vi "AlliGator Load Dataset or Series.vi"(4 "Save Phasor Plot with Overlay":bool, 6 "Save Image with Overlay":bool, 7 "VI in":refnum<vi>, 8 "error in (no error)":errorcluster, 9 "Type of Displayed Image":T1 caption="Displayed Image", 10 "File/Folder Path":path, 11 "AlliGator Ctrl Refnums":T2) -> (0 "error out":errorcluster, 1 "Message":string, 3 "AlliGator Q Elements out":T10[](array[typedef]))   [LabVIEW 2021, in "AlliGator Files.lvlib"]
doc: "Detects type of file loaded and generates the series of actions needed to load it."
uses:
  AlliGator Files.lvlib
  AlliGator Q Element.ctl
  AlliGator Q Event.ctl
  AlliGator Ctrl Refnums.ctl
  AlliGator Other Ctrl Refnums.ctl
  AlliGator State Indicator.ctl
  AlliGator Phasor Plot Ctrl Refnums.ctl
  AlliGator Phasor Graph Ctrl Refnums.ctl
  Phasor/Phasor Calibration Type.ctl
  AlliGator Dataset Ctrl Refnums.ctl
  AlliGator Displayed Image.ctl
  AlliGator Registered Events Ctrl Refnums.ctl
  AlliGator Image Histogram Control Refnums.ctl
  Histograms/Linear Histogram Options.ctl
  Histograms/Histogram Bin Option.ctl
  Histograms/Histogram Bin Position.ctl
  AlliGator Decay Fit Map Control Refnums.ctl
  Fits/IRF(X)PSED/Decay Fit Parameters & Derived Quantities List.ctl
  AlliGator FLI Dataset Type.ctl
  Files/Load-Save File Info.ctl
  AlliGator ROI Manager Actions.ctl
  AlliGator Select Folder Mode.ctl
  AlliGator Folder Selection.ctl
  <vilib>/Utility/error.llb/Error Cluster From Error Code.vi
  AlliGator Source Image ROI Storage [SGL] v3.vi
  <userlib>/_OpenG.lib/array/array.llb/Filter 1D Array with Scalar (String)__ogtk.vi
  <vilib>/ErrorRing/Error Ring.xnode
  AlliGator HDF5.lvlib
  <userlib>/_OpenG.lib/file/file.llb/openg_file.lvlib
  Files/Files.lvlib
  Image/Image.lvlib
  AlliGator Action Engine.lvlib
  <userlib>/_OpenG.lib/array/array.llb/openg_array.lvlib
  AlliGator ROIs.lvlib
  Graphs/XY Graph/XY Graph Add-Ons.lvlib
  AlliGator Globals, Variables & Constants.lvlib
  AlliGator Scripts.lvlib
  AlliGator Decay Fit Parameter Map.lvlib
  GUI/GUI.lvlib
  AlliGator Settings.lvlib
  Sound/Sound.lvlib
  AlliGator Source Image.lvlib
  AlliGator GUI.lvlib
  Phasor/Phasor.lvlib
  Histograms/Histogram Window.lvlib
  Fits/Fits.lvlib
panel:
  out "Script out":bool
  in  "Script in":bool
  # "see the AlliGator License on the block diagram (Ctrl+E or Window:Show Block Diagram)"
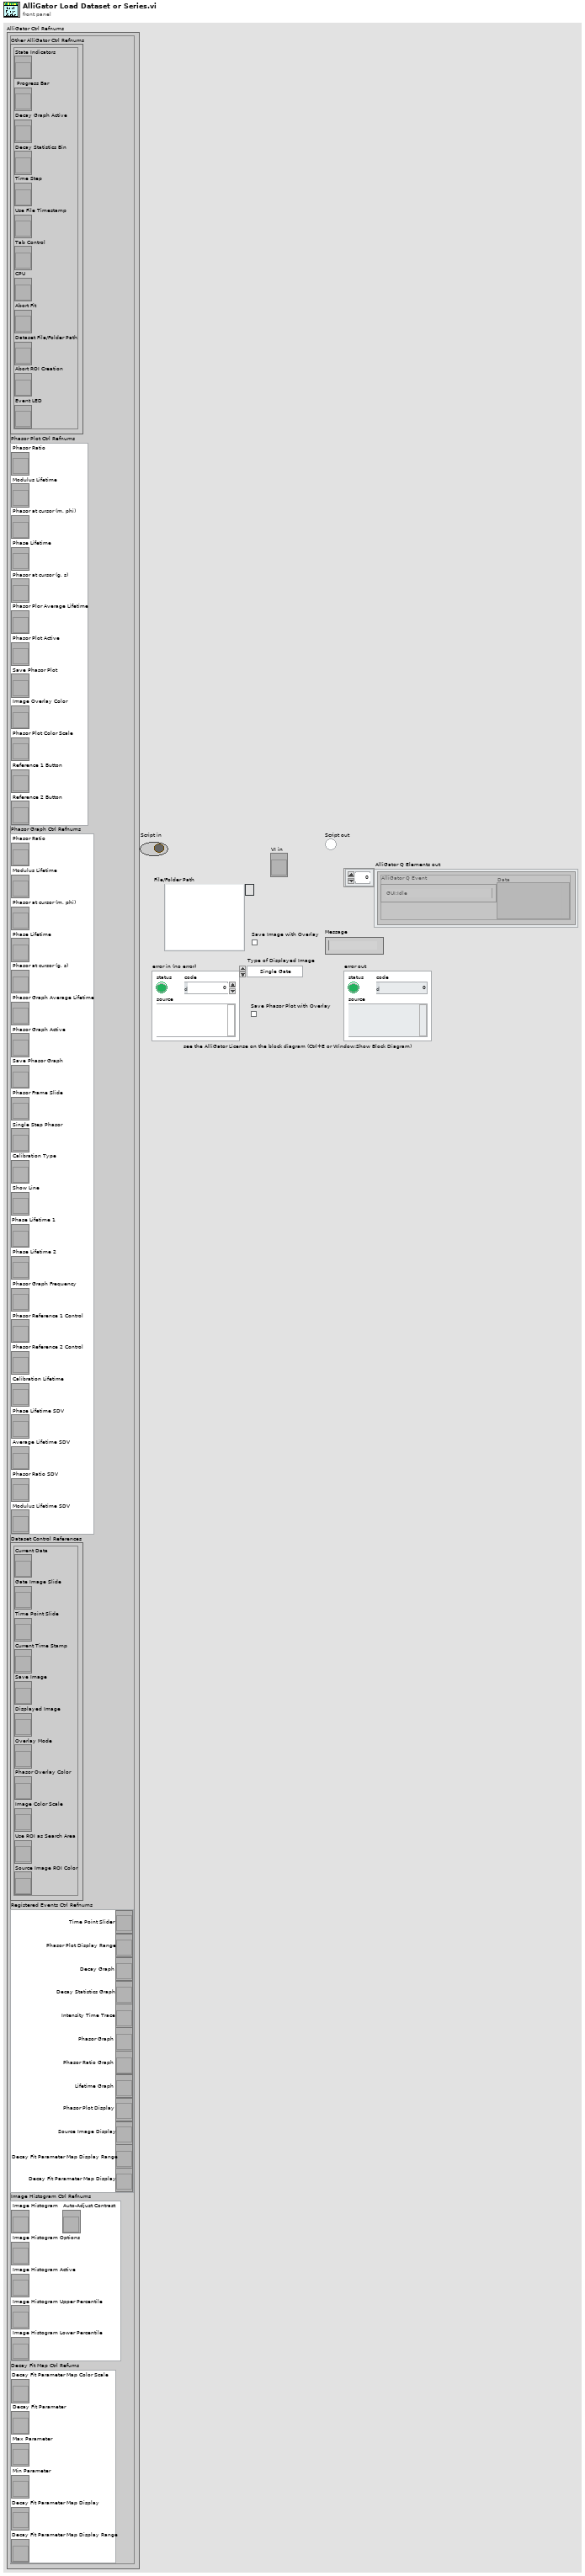
[diagram p1: front panel]
types:
  T1 = typedef "AlliGator Source Image.lvlib/AlliGator Displayed Image.ctl" = enum16{"Single Gate", "Sum of All Gates", "Max of All Gates", "Min of All Gates", "-", "White Ligth Image", "Mask Image"}
  T2 = typedef "AlliGator GUI.lvlib/AlliGator Ctrl Refnums.ctl" = cluster{"Other AlliGator Ctrl Refnums":T3, "Phasor Plot Ctrl Refnums":T4, "Phasor Graph Ctrl Refnums":T5, "Dataset Control References":T6, "Registered Events Ctrl Refnums":T7, "Image Histogram Ctrl Refnums":T8, "Decay Fit Map Ctrl Refums":T9}
  T3 = typedef "AlliGator GUI.lvlib/AlliGator Other Ctrl Refnums.ctl" = cluster{"State Indicators":refnum<vi>, " Progress Bar":refnum<vi>, "Decay Graph Active":refnum<vi>, "Decay Statistics Bin":refnum<vi>, "Time Step":refnum<vi>, "Use File Timestamp":refnum<vi>, "Tab Control":refnum<vi>, "CPU":refnum<vi>, "Abort Fit":refnum<vi>, "Dataset File/Folder Path":refnum<vi>, "Abort ROI Creation":refnum<vi>, "Event LED":refnum<vi>}
  T4 = typedef "AlliGator GUI.lvlib/AlliGator Phasor Plot Ctrl Refnums.ctl" = cluster{"Phasor Ratio":refnum<vi>, "Modulus Lifetime":refnum<vi>, "Phasor at cursor (m, phi)":refnum<vi>, "Phase Lifetime":refnum<vi>, "Phasor at cursor (g, s)":refnum<vi>, "Phasor Plor Average Lifetime":refnum<vi>, "Phasor Plot Active":refnum<vi>, "Save Phasor Plot":refnum<vi>, "Image Overlay Color":refnum<vi>, "Phasor Plot Color Scale":refnum<vi>, "Reference 1 Button":refnum<vi>, "Reference 2 Button":refnum<vi>}
  T5 = typedef "AlliGator GUI.lvlib/AlliGator Phasor Graph Ctrl Refnums.ctl" = cluster{"Phasor Ratio":refnum<vi>, "Modulus Lifetime":refnum<vi>, "Phasor at cursor (m, phi)":refnum<vi>, "Phase Lifetime":refnum<vi>, "Phasor at cursor (g, s)":refnum<vi>, "Phasor Graph Average Lifetime":refnum<vi>, "Phasor Graph Active":refnum<vi>, "Save Phasor Graph":refnum<vi>, "Phasor Frame Slide":refnum<vi>, "Single Step Phasor":refnum<vi>, "Calibration Type":refnum<vi>, "Show Line":refnum<vi>, "Phase Lifetime 1":refnum<vi>, "Phase Lifetime 2":refnum<vi>, "Phasor Graph Frequency":refnum<vi>, "Phasor Reference 1 Control":refnum<vi>, "Phasor Reference 2 Control":refnum<vi>, "Calibration Lifetime":refnum<vi>, "Phase Lifetime SDV":refnum<vi>, "Average Lifetime SDV":refnum<vi>, "Phasor Ratio SDV":refnum<vi>, "Modulus Lifetime SDV":refnum<vi>}
  T6 = typedef "AlliGator GUI.lvlib/AlliGator Dataset Ctrl Refnums.ctl" = cluster{"Current Data":refnum<vi>, "Gate Image Slide":refnum<vi>, "Time Point Slide":refnum<vi>, "Current Time Stamp":refnum<vi>, "Save Image":refnum<vi>, "Displayed Image":refnum<vi>, "Overlay Mode":refnum<vi>, "Phasor Overlay Color":refnum<vi>, "Image Color Scale":refnum<vi>, "Use ROI as Search Area":refnum<vi>, "Source Image ROI Color":refnum<vi>}
  T7 = typedef "AlliGator GUI.lvlib/AlliGator Registered Events Ctrl Refnums.ctl" = cluster{"Time Point Slider":refnum<vi>, "Phasor Plot Display Range":refnum<vi>, "Decay Graph":refnum<vi>, "Decay Statistics Graph":refnum<vi>, "Intensity Time Trace":refnum<vi>, "Phasor Graph":refnum<vi>, "Phasor Ratio Graph":refnum<vi>, "Lifetime Graph":refnum<vi>, "Phasor Plot Display":refnum<vi>, "Source Image Display":refnum<vi>, "Decay Fit Parameter Map Display Range":refnum<vi>, "Decay Fit Parameter Map Display":refnum<vi>}
  T8 = typedef "AlliGator GUI.lvlib/AlliGator Image Histogram Control Refnums.ctl" = cluster{"Image Histogram":refnum<vi>, "Image Histogram Options":refnum<vi>, "Image Histogram Active":refnum<vi>, "Image Histogram Upper Percentile":refnum<vi>, "Image Histogram Lower Percentile":refnum<vi>, "Auto-Adjust Contrast":refnum<vi>}
  T9 = typedef "AlliGator Decay Fit Parameter Map.lvlib/AlliGator Decay Fit Map Control Refnums.ctl" = cluster{"Decay Fit Parameter Map Color Scale":refnum<vi>, "Decay Fit Parameter":refnum<vi>, "Max Parameter":refnum<vi>, "Min Parameter":refnum<vi>, "Decay Fit Parameter Map Display":refnum<vi>, "Decay Fit Parameter Map Display Range":refnum<vi>}
  T10 = typedef "AlliGator Action Engine.lvlib/AlliGator Q Element.ctl" = cluster{"AlliGator Q Event":T11, "Data":variant}
  T11 = typedef "AlliGator Action Engine.lvlib/AlliGator Q Event.ctl" = enum16{"---- Files ----", "Files:Set Batch Export Files To Save", "Files:Set Dataset Loading & Pre-processing Options", "Files:Check #Frames in Dataset", "Files:Increment Frame Index", "Files:Open Mask Image", "Files:Open White Light Image", "Files:Open Single Dataset", "Files:New Folder of Folders Selected", "Files:Load File (all Types)_Scriptable", "Files:Move Flattened Series to Folders Series", "Files:Select Folder", "Files:Load FLI Dataset", "Files:Load Swiss SPAD 1 Dataset", "Files:Load Swiss SPAD 2 Dataset", "Files:Load .sdt FLI Dataset", "Files:Load .ptu FLI Dataset", "Files:Load .bin FLI Dataset", "Files:Load Single Gate Image Folder", "Files:Load I/m/phi Dataset (deprecated)", "Files:Load Single Image", "Files:Subtract Background File", "Files:Export FLI Dataset", "Files:Load HDF5 FLI Dataset", "Files:Set Destination File Path", "Files:Save Mask Image", "Files:Batch Conversion", "Files:New Folder Selected", "Files:Close FLI Dataset", "Files:Close FLI Dataset Series", "Files:Close White Light Image", "Files:Close Mask Image", "---- FLI Dataset ----", "FLI Dataset:Channel Arithmetic", "FLI Dataset:Export Average Lifetime Map as ASCII", "FLI Dataset:Export User-Defined Quantity Map as ASCII", "FLI Dataset:Python Function FLI Dataset Event", "FLI Dataset:ROI Analysis", "FLI Dataset:Tilted Logistic Square Gated IRF Characteristics Map", "FLI Dataset:Logistic Square Gated IRF Characteristics Map", "FLI Dataset:Square Gated IRF Characteristics Map", "FLI Dataset:Multi-ROI Single-Pixel Phasor Analysis", "FLI Dataset:Multi-ROI Single-Pixel NLSF Analysis", "FLI Dataset:All ROIs IRF Extraction", "FLI Dataset:All ROIs Decay Fit Non-Interactive (Fast + Individual IRF)", "FLI Dataset:All ROIs Phasor Analysis", "FLI Dataset:All ROIs Decay Fit", "FLI Dataset:Fluorescence Decay Statistics", "FLI Dataset:Update Decay Statistics Graph", "FLI Dataset:Get Decay from ROI", "FLI Dataset:All ROIs Average Lifetimes", "---- FLI Dataset Series ----", "FLI Dataset Series:Sum All Datasets in Series", "FLI Dataset Series:Add Dataset to Accumulated Dataset", "FLI Dataset Series:Display Accumulated Dataset", "FLI Dataset Series:Clear Dataset Series Sum", "FLI Dataset Series:Time-Series Analysis (NLSF)", "FLI Dataset Series:Time-Series Analysis (Phasor)", "---- Image ----", "Image:Update Image Profile Plots", "Image:Image Histogram Cursor Move", "Image:Image Histogram", "Image:Image Contrast", "Image:Set Image Histogram Cursor Move Flag", "Image:Clear Image Overlay", "Image:Use ROI as Search Area", "Image:Set ROI Diameter", "Image:Save Image Data as TIFF", "Image:Save Displayed Image with Overlay", "Image:Save Image Overlay Only", "Image:Save Image as Hot Pixel Mask", "Image:Change Source Image Color Palette", "Image:Copy Image to Clipboard", "Image:Source Image ROI Selection", "Image:Delete All ROIs", "Image:Delete All Unselected ROIs", "Image:Delete ROI", "Image:Merge All ROIs", "Image:Store ROI", "Image:Source Image ROI Storage", "Image:Export ROI Description to Notebook", "Image:Save ROI", "Image:Load ROI", "Image:Paste ROI Definition", "Image:Clear ROI", "Image:Identify ROIs in Mask Image", "Image:Create Complementary ROI", "Image:Create Contour ROI", "Image:Create ROI(s) from Pixels with Peak above Min_Scriptable", "Image:Create ROI(s) from Pixels with Intensity above Min_Scriptable", "Image:Compute ROI Statistics", "Image:Delete ROI(s) based on ROI Characteristics", "Image:Create ROI Grid", "Image:ROI to Individual Pixel ROIs", "Image:Python Function Source Image Event", "Image:Show Phasor Calibration Map ROI Centers", "Image:Convert ROI to Mask Image", "Image:Mouse Move", "Image:Mouse Up", "Image:Set Source Image Mouse Move Flag", "Image:Add Scale Bar Overlay", "Image:Delete Existing ROIs Option", "---- Decay ----", "Decay:Clear IRF/Reference Plot", "Decay:Clear Local IRFs", "Decay:Add Decay to Graph", "Decay:Smoothen Plot", "Decay:Smoothen Plot Tail", "Decay:Average Selected Plots", "Decay:Extract IRF", "Decay:Optimal IRF Extraction", "Decay:Threshold IRF", "Decay:Fit to Model IRF", "Decay:Fit IRF to Square Gate", "Decay:Fit IRF to Logistic Square Gate", "Decay:Fit IRF to Tilted Logistic Square Gate", "Decay:Create Bounding Cursors Set", "Decay:Export Bounding Cursors Definition to Notebook", "Decay:Denoise Plot", "Decay:Compute Cumulative Function", "Decay:Use as Reference Decay", "Decay:Show Reference Decay/IRF", "Decay:Extrapolate Decay", "Decay:Create Head & Tail Bounding Cursors", "Decay:Store Cursor-defined Head & Tail Fractions", "Decay:Rebin Plot", "Decay:1-Normalize Decay", "Decay:[0-1]-Normalize Plot", "Decay:Straighten Decay", "Decay:Shift Decay", "Decay:Fold Decay", "Decay:Fit Decay", "Decay:Global Fit of Selected Decays", "Decay:Post Global Fit Script", "Decay:Add Global Fit Parameters to Graph", "Decay:Add Decay Parameter(s) to Plot (Graph)", "Decay:Export Decay to Phasor Graph", "Decay:Plot Decay Shifts", "Decay:Compute Average Lifetime", "Decay:Plot Convolution", "Decay:Graph Tip Strip Update", "---- Decay Statistics ----", "Decay Statistics:Tip Strip Update", "---- Intensity Time Trace ----", "Intensity Time Trace:Use File Timestamp", "Intensity Time Trace:Load Intensity Corrections File", "Intensity Time Trace:Clear Intensity Corrections File", "Intensity Time Trace:Tip Strip Update", "---- Phasor Plot ----", "Phasor Plot:Build Phasor Plot", "Phasor Plot:Change Phasor Plot Color Palette", "Phasor Plot:Adjust Phasor Plot Display Range", "Phasor Plot:Highlight Image ROI in Phasor Plot", "Phasor Plot:Save Phasor Plot Image with Overlay", "Phasor Plot:Export Complex Phasor Map", "Phasor Plot:Export Phasor Ratio Map", "Phasor Plot:Export Average Lifetime Map", "Phasor Plot:Compute Phase Lifetime Histogram", "Phasor Plot:Compute Phasor Ratio Histogram", "Phasor Plot:Compute Phase Lifetime vs Intensity Scatter Plot", "Phasor Plot:Weber 2-Component Decomposition", "Phasor Plot:Update Phasor Color Map Vertices", "Phasor Plot:Clear Phasor Overlay", "Phasor Plot:Use Segment Extremities as References", "Phasor Plot:Use UC/Segment Intersections as References", "Phasor Plot:Use UC/Principal Axis Intersections as References", "Phasor Plot:Use UC/Linear Fit Intersections as References", "Phasor Plot:Update Phasor Plot Reference", "Phasor Plot:Show Local Phasor Info in Phasor Plot", "Phasor Plot:Update Phasor Plot State", "Phasor Plot:Phasor Plot ROI Storage", "Phasor Plot:Phasor Plot ROI Selection", "Phasor Plot:Python Function Phasor Plot Event", "Phasor Plot:Overlay Phasor ROI, Ratio or Map in Source Image", "Phasor Plot:Compute Decay of Selected Phasors", "Phasor Plot:Phasor at Image Pixel", "Phasor Plot:Mouse Move", "Phasor Plot:Mouse Up", "Phasor Plot:Display Range Mouse Move", "Phasor Plot:Set Mouse Move Flag", "---- Phasor Graph ----", "Phasor Graph:Calibrated Phasor Map Series", "Phasor Graph:Whole Image Phasor Scatter Plot (Todo)", "Phasor Graph:Get Phasor Value", "Phasor Graph:Create New Phasor Plot Dialog", "Phasor Graph:Update Last Phasor Value", "Phasor Graph:Update Phasor (m, phi)", "Phasor Graph:Remove Single Phasor from Plot", "Phasor Graph:Add Single Phasor to Plot", "Phasor Graph:Remove Phasor Plot", "Phasor Graph:Remove Selected Phasor Plots", "Phasor Graph:Clear Phasor Data", "Phasor Graph:Clear Phasor Graph", "Phasor Graph:Cursor Move", "Phasor Graph:Draw Cursor Connecting Line", "Phasor Graph:Clear Cursor Connecting Line", "Phasor Graph:Find UC Intersection", "Phasor Graph:Use UC/Cursor-Defined Line Intersections", "Phasor Graph:Use Selected Plots Fitted Line/UC Intersections", "Phasor Graph:Use Selected Plots Principal Axis/UC Intersections", "Phasor Graph:Show Single Phasor", "Phasor Graph:Save Single Phasor Plot", "Phasor Graph:Save All Phasor Plots", "Phasor Graph:Load Phasor Plot(s)", "Phasor Graph:Phasor Multiplication", "Phasor Graph:Compute Average Phasor", "Phasor Graph:Compute Multiple Average Phasors (Selected Plots)", "Phasor Graph:Export Single Phasor Plot Phase Lifetimes", "Phasor Graph:Phase Lifetime Trajectory", "Phasor Graph:Phase Lifetime vs Intensity Scatter Plot (deprecated)", "Phasor Graph:Parameter 2 vs Parameter 1 Scatter Plot", "Phasor Graph:Use Cursor n Location", "Phasor Graph:Set Reference n to Current Phase Lifetime Value", "Phasor Graph:Set Reference n to Lifetime Value", "Phasor Graph:Set Cursor n Location", "Phasor Graph:Save Phasor Graph Image", "Phasor Graph:Update SEPL Plot", "Phasor Graph:Export Single Phasor Plot Data", "Phasor Graph:Export Selected Phasor Plots Data", "Phasor Graph:Python Function Phasor Graph Event", "Phasor Graph:Tip Strip Update", "---- Calibration ----", "Calibration:Set Calibration Type", "Calibration:Load/Save Phasor Calibration", "Calibration:Load/Save Phasor Calibration Series", "Calibration:Load/Save Phasor Calibration Map", "Calibration:Use as Calibration", "Calibration:Compute Optimal Calibration from Phasor References", "Calibration:Clear Phasor Calibration", "Calibration:Use as Calibration Series", "Calibration:Use as Calibration Map", "Calibration:Clear Calibration Series", "Calibration:Clear Calibration Map", "Calibration:Apply Phasor Calibration", "Calibration:Update Single Plot Calibration", "Calibration:Update Multiple Plots Calibration", "Calibration:Clear Single Plot Calibration", "Calibration:Clear All Plots Calibrations", "Calibration:Clear Plot(s) Calibration(s)?", "Calibration:Phasor Calibration Maps (# Gates Series)", "---- Phasor Ratio ----", "Phasor Ratio:Clear Reference n", "Phasor Ratio:Toggle Selected Plot(s)  Lock to Reference 1", "Phasor Ratio:Use as Reference n", "Phasor Ratio:Send Reference n to Notebook", "Phasor Ratio:Toggle Selected Plot(s)  Lock to Reference 2", "Phasor Ratio:Compute Phasor Ratio at Mouse Location", "Phasor Ratio:Compute Phasor Plot's Average Phasor Ratio", "Phasor Ratio:Compute Time-Series Phasor Ratios", "Phasor Ratio:Fit Line to Phasor Ratio Plot", "Phasor Ratio:Save References", "Phasor Ratio:Load References", "Phasor Ratio:Update Phasor Reference 1", "Phasor Ratio:Update Phasor Reference 2", "Phasor Ratio:Move Cursor n to Reference n", "Phasor Ratio:Use as Phasor Reference 1 Lifetime", "Phasor Ratio:Use as Phasor Reference 2 Lifetime", "Phasor Ratio:Export Phasor Ratio Map as ASCII", "Phasor Ratio:Tip Strip Update", "---- Lifetime & Other Parameters Graph ----", "Lifetime:Tip Strip Update", "---- Decay Fit Parameter Map ----", "Decay Fit Parameter Map:Export ROI NLSF Data as ASCII", "Decay Fit Parameter Map:Set Decay Fit  Parameter Map Selection", "Decay Fit Parameter Map:Build Decay Fit Parameter Map", "Decay Fit Parameter Map:Change Decay Fit Parameter Map Color Palette", "Decay Fit Parameter Map:Export Decay Fit Parameter Map Data as ASCII", "Decay Fit Parameter Map:Export All Decay Fit Parameter Maps Data as ASCII", "Decay Fit Parameter Map:Send Map Data to Lifetime Graph", "Decay Fit Parameter Map:Save Decay Fit Parameter Map Image", "Decay Fit Parameter Map:Save-Load IRFs & Fit Data", "Decay Fit Parameter Map:Update Local Decay Plots", "Decay Fit Parameter Map:Python Function Decay Fit Parameters Map Event", "Decay Fit Parameter Map:Overlay Decay Fit Parameter Map in Source Image", "Decay Fit Parameter Map:Plot Map Data vs Intensity", "Decay Fit Parameter Map:Mouse Up", "Decay Fit Parameter Map:Display Range Mouse Move", "---- Generic Graph ----", "Generic Graph:Generic XY Graph Event", "Generic Graph:Python Function XY Graph Event", "Generic Graph:New Plot", "Generic Graph:Save Plot", "Generic Graph:XY Plot Histogram", "Generic Graph:Set XY Graph Plot Name", "Generic Graph:Set Last Cursor Style", "Generic Graph:Tip Strip Update", "---- GUI ----", "GUI:Start Script", "GUI:Type of Displayed Image Changed", "GUI:Gate Image Slide Changed", "GUI:Show Busy Icon", "GUI:Show Busy Icon & Abort Button", "GUI:Hide Busy Icon", "GUI:Hide Busy Icon & Abort Button", "GUI:Abort", "GUI:End Script", "GUI:Start Timing", "GUI:End Timing", "GUI:Set State Indicator", "GUI:Send Parameters JSON Strings to Clipboard", "GUI:Set Gate Step", "GUI:Idle", "GUI:Initialization", "GUI:Quit", "GUI:Increment Dataset Index", "GUI:Set Dataset Index to -1", "GUI:Time Series Slider Moved", "GUI:Time Series Slider Changed", "GUI:Toggle Playback or Loop", "GUI:Playback Script", "GUI:Set Phasor Frequency", "GUI:Open Window", "DEBUG"}
  T12 = typedef "AlliGator Files.lvlib/AlliGator FLI Dataset Type.ctl" = enum16{"HDF5 FLI Dataset", "Gate Image Folder", ".sdt FLI Dataset (Becker & Hickl)", ".ptu FLI Dataset (PicoQuant)", "SS1 FLI Dataset", "SS2 FLI Dataset", "I/m/phi Dataset", ".bin FLI Dataset (PicoQuant Binned)", ".bin FLI Dataset (Piccolo Binned)"}
  T13 = typedef "Files.lvlib/Load-Save File Info.ctl" = cluster{"Load/Save":bool, "File Path":path}
  T14 = typedef "ROI Descriptor" = cluster{"Global Rectangle":i32[], "Contours":cluster{"ID":enum32{"External", "Internal"}, "Type":u32, "Coordinates":i32[]}[]}
  T15 = typedef "AlliGator ROIs.lvlib/AlliGator ROI Manager Actions.ctl" = enum16{"Undefined", "Delete Current ROI", "Delete All Unselected ROIs", "Delete Multiple ROIs", "Delete All ROIs", "Swap ROIs", "Insert ROI", "Update Current ROI Descriptor", "Rename Current ROI", "Store New ROI", "Store Multiple ROIs", "Select Next ROI", "Select Previous ROI", "Find Selected ROI", "Show All ROIs", "Update ROI Manager Window", "Merge All ROIs", "Unmerge ROI", "Set Selected ROI by ID"}
  T16 = typedef "AlliGator Files.lvlib/AlliGator Folder Selection.ctl" = cluster{"Folder Selection Mode":T17, "Folder Path":path}
  T17 = typedef "AlliGator Files.lvlib/AlliGator Select Folder Mode.ctl" = enum16{"Select Gate Folder", "Select Folder of Gate Folders", "Select Folder of SwissSPAD 2 Datasets", "Select Folder of .sdt FLI Datasets (Becker & Hickl)", "Select Folder of .ptu FLI Datasets (PicoQuant)", "Select Folder of .bin FLI Datasets (PicoQuant Binned)", "Select Folder of .bin FLI Datasets (Piccolo Binned)", "Select Folder of HDF5 FLI Datasets"}
  T18 = typedef "Image Type" = u32
  T19 = typedef "Fits.lvlib/3-Button Dialog Output.ctl" = enum16{"Window Close", "Button 1", "Button 2", "Button 3"}
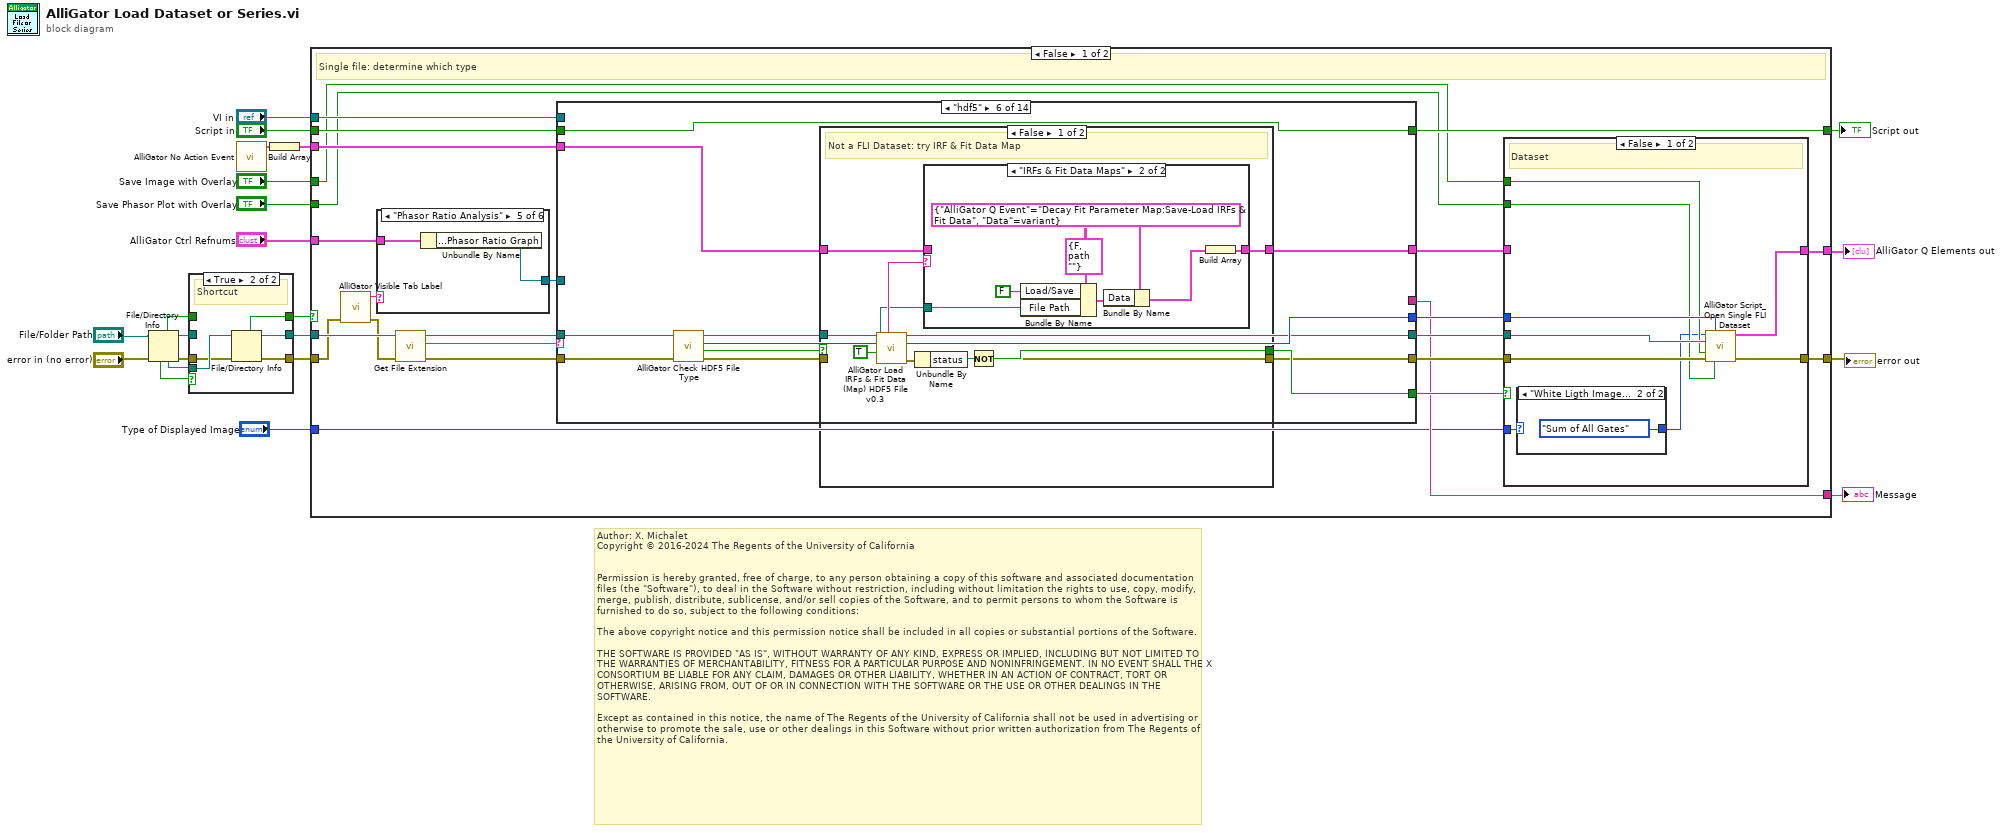
[diagram p0: block diagram]
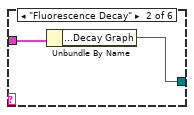
[diagram p3: hidden frame]
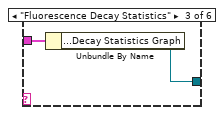
[diagram p4: hidden frame]
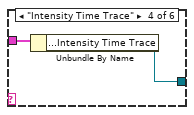
[diagram p5: hidden frame]
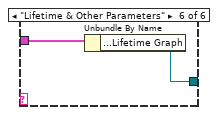
[diagram p6: hidden frame]
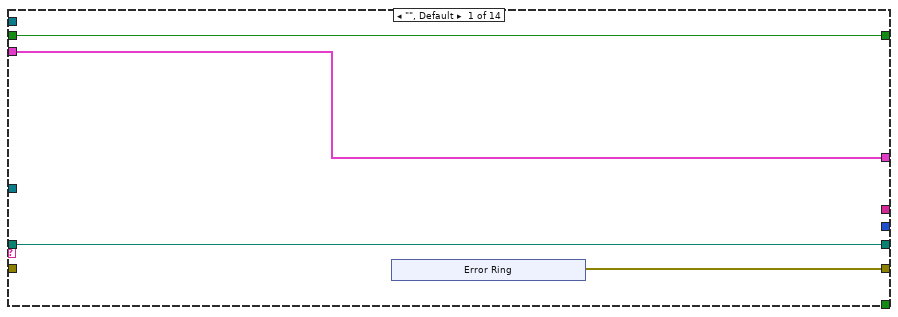
[diagram p9: hidden frame]
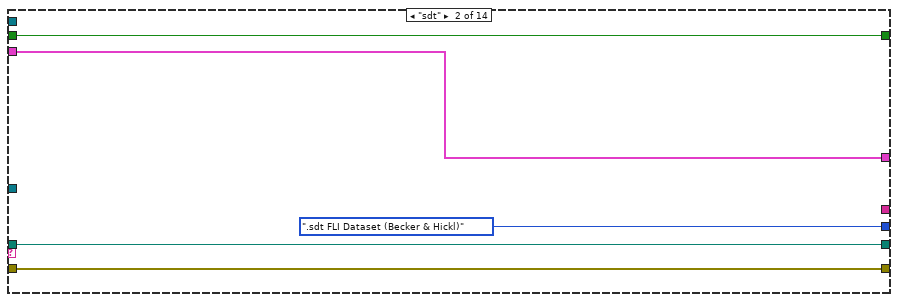
[diagram p10: hidden frame]
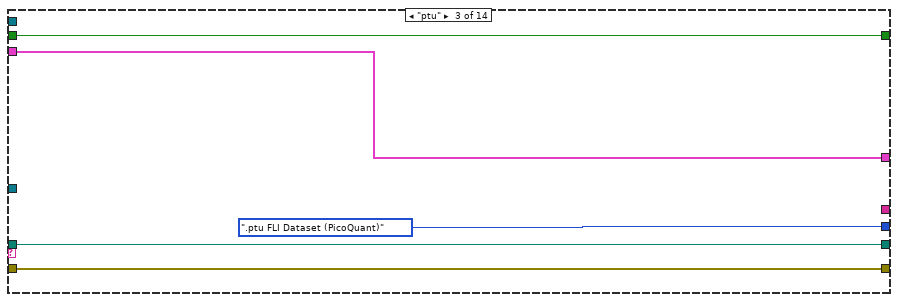
[diagram p11: hidden frame]
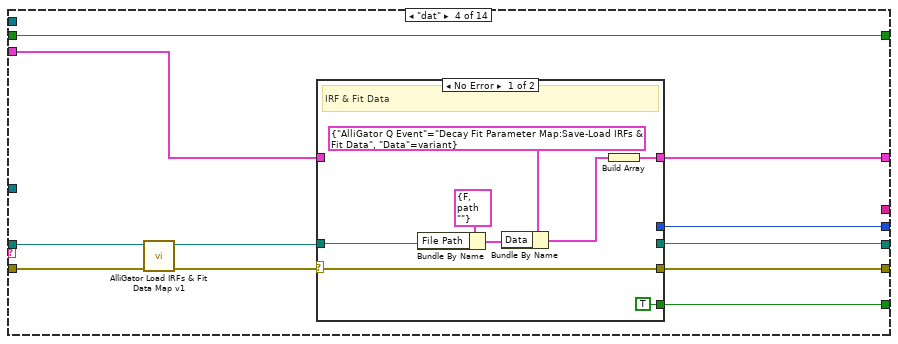
[diagram p12: hidden frame]
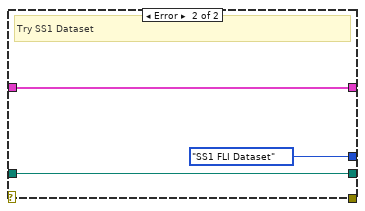
[diagram p13: hidden frame]
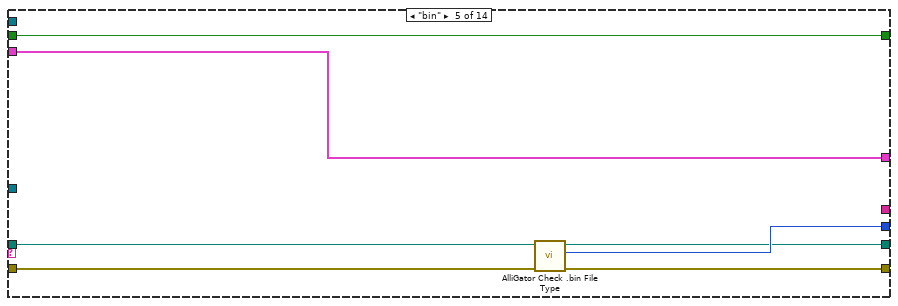
[diagram p14: hidden frame]
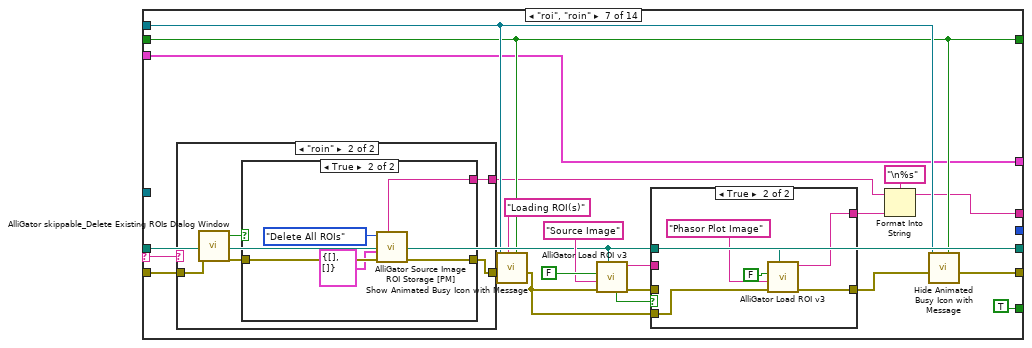
[diagram p17: hidden frame]
diagram:
  # "Author: X. Michalet\nCopyright © 2016-2024 The Regents of the University of California\n \n\nPermission is hereby granted, free of charge, to any person obtaining a copy of this software and associated documentation files (the \"Software\"), to deal in the Software without restriction, including without limitation the rights to use, copy, modify, merge, publish, distribute, sublicense, and/or sell copies of the Software, and to permit persons to whom the Software is furnished to do so, subject to the following conditions:\n\nThe above copyright notice and this permission notice shall be included in all copies or substantial portions of the Software.\n\nTHE SOFTWARE IS PROVIDED \"AS IS\", WITHOUT WARRANTY OF ANY KIND, EXPRESS OR IMPLIED, INCLUDING BUT NOT LIMITED TO THE WARRANTIES OF MERCHANTABILITY, FITNESS FOR A PARTICULAR PURPOSE AND NONINFRINGEMENT. IN NO EVENT SHALL THE X CONSORTIUM BE LIABLE FOR ANY CLAIM, DAMAGES OR OTHER LIABILITY, WHETHER IN AN ACTION OF CONTRACT, TORT OR OTHERWISE, ARISING FROM, OUT OF OR IN CONNECTION WITH THE SOFTWARE OR THE USE OR OTHER DEALINGS IN THE SOFTWARE.\n\nExcept as contained in this notice, the name of The Regents of the University of California shall not be used in advertising or otherwise to promote the sale, use or other dealings in this Software without prior written authorization from The Regents of the University of California."
  n1 = File/Directory Info(path="File/Folder Path", error in="error in (no error)") -> (path out=w16:path, directory=w13:bool, error out=w15:errorcluster, resolved path=w17:path, shortcut=w18:bool)  [unwired: 2 out]
  n2 = case shown="True" w18 {
    tunnel: w17 -> [_ w30]
    tunnel: w16 -> [w24 _]
    tunnel: w15 -> [w23 w29]
    tunnel: [w25 w28] -> w14
    tunnel: w13 -> [w25 _]
    tunnel: [w24 w27] -> w12
    tunnel: [w23 w26] -> w11
    frame False {
      # "not a shortcut"
    }
    frame True {
      # "Shortcut"
      n3 = File/Directory Info(path=w30, error in=w29) -> (path out=w27:path, directory=w28:bool, error out=w26:errorcluster)  [unwired: 4 out]
    }
  }
  n4 = call "AlliGator No Action Event.vi"() -> ("No Action"=w7:T10)
  n5 = Build Array(w7) -> (w6:T10[])
  n6 = case shown="False" w14 {
    tunnel: w12 -> [w54 w301]
    tunnel: w11 -> [w45 w300]
    tunnel: [w41 w299] -> w20
    tunnel: [w50 w295] -> w19
    tunnel: "Save Image with Overlay" -> [w32 w292]
    tunnel: "Save Phasor Plot with Overlay" -> [w31 w291]
    tunnel: "AlliGator Ctrl Refnums" -> [w40 _]
    tunnel: w6 -> [w39 _]
    tunnel: [w37 _] -> w5
    tunnel: "VI in" -> [w36 _]
    tunnel: "Script in" -> [w35 w290]
    tunnel: [w34 w290] -> w2
    tunnel: "Type of Displayed Image" -> [w33 w289]
    frame False {
      # "Single file: determine which type"
      n7 = call "AlliGator Visible Tab Label.vi"("Error In"=w45) -> ("Error Out"=w42:errorcluster, "Visible Tab"=w44:string)  [unwired: 9 in]
      n8 = case shown="\"Phasor Ratio Analysis\"" w44 {
        tunnel: [_ w55 w57 w59 w61 w63] -> w43
        tunnel: w40 -> [_ w56 w58 w60 w62 w64]
        frame "", Default {
        }
        frame "Fluorescence Decay" {
          n9 = Unbundle By Name(w56) -> ("Registered Events Ctrl Refnums.Decay Graph"=w55:refnum<vi>)
        }
        frame "Fluorescence Decay Statistics" {
          n10 = Unbundle By Name(w58) -> ("Registered Events Ctrl Refnums.Decay Statistics Graph"=w57:refnum<vi>)
        }
        frame "Intensity Time Trace" {
          n11 = Unbundle By Name(w60) -> ("Registered Events Ctrl Refnums.Intensity Time Trace"=w59:refnum<vi>)
        }
        frame "Phasor Ratio Analysis" {
          n12 = Unbundle By Name(w62) -> ("Registered Events Ctrl Refnums.Phasor Ratio Graph"=w61:refnum<vi>)
        }
        frame "Lifetime & Other Parameters" {
          n13 = Unbundle By Name(w64) -> ("Registered Events Ctrl Refnums.Lifetime Graph"=w63:refnum<vi>)
        }
      }
      n14 = call <vilib>:"Get File Extension.vi"("error in (no error)"=w42, "file"=w54) -> ("error out"=w52:errorcluster, "lowercase file extension"=w53:string, "dup file"=w49:path)  [unwired: 5 in, 2 out]
      n15 = case shown="\"hdf5\"" w53 {
        selector: w53 -> [_ _ _ _ _ _ w160 _ _ _ _ _ _ _]
        tunnel: w52 -> [_ w89 w94 w102 w120 w134 w159 w199 w214 w249 w258 w266 w275 w285]
        tunnel: [w81 w89 w94 w104 w119 w128 w166 w202 w209 w249 w258 w266 w275 w285] -> w51
        tunnel: [_ AlliGator_FLI_Dataset_Type.".sdt FLI Dataset (Becker & Hickl)" ("FLI Dataset Type") AlliGator_FLI_Dataset_Type.".ptu FLI Dataset (PicoQuant)" ("FLI Dataset Type") w106 w124 w133 _ _ _ _ _ _ _ _] -> w47
        tunnel: w49 -> [w80 w88 w93 w101 w121 w135 w170 w204 w211 w253 w259 w268 w277 w282]
        tunnel: [w80 w88 w93 w98 w118 w130 w170 w204 _ _ _ _ _ _] -> w48
        tunnel: [_ _ _ w103 _ w131 TRUE TRUE TRUE TRUE TRUE TRUE TRUE TRUE] -> w46
        tunnel: w43 -> [_ _ _ _ _ _ _ w203 _ _ _ _ _ _]
        tunnel: [w79 w87 w92 w105 w123 w127 w161 w198 w210 w248 w256 w265 w274 w284] -> w38
        tunnel: w39 -> [w79 w87 w92 w97 w123 w126 w161 w198 w208 _ _ _ _ _]
        tunnel: [_ _ _ _ _ _ w156 w197 _ _ _ _ _ _] -> w37
        tunnel: w36 -> [_ _ _ _ _ _ w165 _ _ _ _ _ _ _]
        tunnel: w35 -> [w78 w86 w91 w96 w122 w125 w162 w195 w207 w247 w255 w264 w273 w283]
        tunnel: [w78 w86 w91 w96 w122 w125 w162 w195 w207 w247 w255 w264 w273 w283] -> w34
        frame "", Default {
          n16 = xnode "Error Ring"() -> ("error out"=w81:errorcluster)
        }
        frame "sdt" {
        }
        frame "ptu" {
        }
        frame "dat" {
          n17 = call "AlliGator Load IRFs & Fit Data Map v1.vi"("error in (no error)"=w102, "File Path in"=w101) -> ("error out"=w99:errorcluster, "File Path out"=w100:path)  [unwired: 7 in, 1 out]
          n18 = case shown="No Error" w99 {
            selector: w99 -> [w108 _]
            tunnel: [_ AlliGator_FLI_Dataset_Type."SS1 FLI Dataset" ("FLI Dataset Type")] -> w106
            tunnel: [w107 w115] -> w105
            tunnel: [w108 _] -> w104
            tunnel: [TRUE _] -> w103
            tunnel: w100 -> [w110 w116]
            tunnel: [_ w116] -> w98
            tunnel: w97 -> [_ w115]
            frame No Error {
              # "IRF & Fit Data"
              n19 = Bundle By Name(cluster=T13 {"Load/Save"=FALSE, "File Path"=path ""}, "File Path"=w110) -> (w114:T13)
              n20 = Bundle By Name(cluster=T10 {"AlliGator Q Event"=enum."Decay Fit Parameter Map:Save-Load IRFs & Fit Data", "Data"=variant} ("Alligator Atomic Action"), "Data"=w114) -> (w109:T10)
              n21 = Build Array(w109) -> (w107:T10[])
            }
            frame Error {
              # "Try SS1 Dataset"
            }
          }
        }
        frame "bin" {
          n22 = call "AlliGator Check .bin File Type.vi"("error in (no error)"=w120, "File Path"=w121) -> ("error out"=w119:errorcluster, "bin FLI Dataset Type"=w124:T12, "File Path dup"=w118:path)  [unwired: 6 in, 1 out]
        }
        frame "hdf5" {
          n23 = call "AlliGator Check HDF5 File Type.vi"("error in (no error)"=w134, "HDF5 File Path in"=w135) -> ("error out"=w129:errorcluster, "FLI Dataset?"=w132:bool, "FLI Dataset Type"=w133:T12, "HDF5 File Path out"=w130:path)  [unwired: 6 in]
          n24 = case shown="False" w132 {
            tunnel: [w141 _] -> w131
            tunnel: w130 -> [w137 _]
            tunnel: w129 -> [_ w153]
            tunnel: [w140 w153] -> w128
            tunnel: [w138 w152] -> w127
            tunnel: w126 -> [w136 w152]
            frame False {
              # "Not a FLI Dataset: try IRF & Fit Data Map"
              n25 = call "AlliGator Load IRFs & Fit Data (Map) HDF5 File v0.3.vi"("File Type & Version only"=TRUE, "File Path"=w137) -> ("error out"=w140:errorcluster, "File Type"=w139:string)  [unwired: 3 in, 5 out]
              n26 = Unbundle By Name(w140) -> ("status"=w142:bool)
              n27 = case shown="\"IRFs & Fit Data Maps\"" w139 {
                tunnel: [w144 w145] -> w138
                tunnel: w137 -> [_ w147]
                tunnel: w136 -> [w144 _]
                frame "", Default {
                }
                frame "IRFs & Fit Data Maps" {
                  n28 = Bundle By Name(cluster=T13 {"Load/Save"=FALSE, "File Path"=path ""} ("Calibration File Information"), "Load/Save"=FALSE, "File Path"=w147) -> (w149:T13)
                  n29 = Bundle By Name(cluster=T10 {"AlliGator Q Event"=enum."Decay Fit Parameter Map:Save-Load IRFs & Fit Data", "Data"=variant} ("Alligator Atomic Action"), "Data"=w149) -> (w146:T10)
                  n30 = Build Array(w146) -> (w145:T10[])
                }
              }
              n31 = Not(x=w142) -> (.not. x?=w141:bool)
            }
            frame True {
              # "FLI Dataset"
            }
          }
        }
        frame "roi", "roin" {
          n32 = case shown="\"roin\"" w160 {
            tunnel: w159 -> [w175 w179]
            tunnel: [w175 w177] -> w158
            tunnel: [_ w176] -> w155
            frame "roi", Default {
            }
            frame "roin" {
              n33 = call "AlliGator skippable_Delete Existing ROIs Dialog Window.vi"("Error In"=w179) -> ("Error Out"=w178:errorcluster, "Delete"=w180:bool)  [unwired: 9 in]
              n34 = case shown="True" w180 {
                tunnel: w178 -> [w181 w186]
                tunnel: [w181 w184] -> w177
                tunnel: [_ w183] -> w176
                frame False {
                }
                frame True {
                  n35 = call-poly "AlliGator Source Image ROI Storage [PM].vi"("Error In"=w186, "Current ROI Descriptor"=T14 {"Global Rectangle"=[], "Contours"=[]}, "Action"=AlliGator_ROI_Manager_Actions."Delete All ROIs") -> ("Error Out"=w184:errorcluster, "Message"=w183:string)  [unwired: 2 in, 5 out]
                }
              }
            }
          }
          n36 = call "Show Animated Busy Icon with Message.vi"("Already active? (F)"=w162, "Message"="Loading ROI(s)", "Error In"=w158, "Target VI Refnum"=w165) -> ("Error Out"=w167:errorcluster)  [unwired: 7 in]
          n37 = call "AlliGator Load ROI v3.vi"("File Path"=w170, "Error In"=w167, "Destination Image (Source Image)"="Source Image" ("Destination Image"), "Dialog (T)"=FALSE) -> ("Error Out"=w168:errorcluster, "Message"=w163:string, "Phasor Plot Image"=w171:bool)  [unwired: 1 in, 4 out]
          n38 = case shown="True" w171 {
            tunnel: w167 -> [_ w194]
            tunnel: w170 -> [_ w192]
            tunnel: [w188 w190] -> w169
            tunnel: w168 -> [w188 _]
            tunnel: [w187 w189] -> w157
            tunnel: w163 -> [w187 _]
            frame False {
            }
            frame True {
              n39 = call "AlliGator Load ROI v3.vi"("File Path"=w192, "Error In"=w194, "Destination Image (Source Image)"="Phasor Plot Image" ("Destination Image"), "Dialog (T)"=FALSE) -> ("Error Out"=w190:errorcluster, "Message"=w189:string)  [unwired: 1 in, 5 out]
            }
          }
          n40 = Format Into String(format string="\n%s", initial string=w155, w157) -> (resulting string=w156:string)  [unwired: 1 in, 1 out]
          n41 = call "Hide Animated Busy Icon with Message.vi"("Already active? (F)"=w162, "Error In"=w169, "Target VI reference"=w165) -> ("Error Out"=w166:errorcluster)  [unwired: 8 in]
        }
        frame "txt" {
          # "Clears Error if visible Graph does not accept loading ASCII plots (e.g. Image Histogram, Phasor Graph)"
          n42 = call "AlliGator Gate Separation (ns).vi"("error in (no error)"=w199) -> ("error out"=w196:errorcluster)  [unwired: 9 in, 1 out]
          n43 = call "XY Graph Load Plot(s) Event.vi"("Error In"=w196, "File Path"=w204, "Used Dialog? (T)"=FALSE ("Dialog (T)"), "XYGraph Ref"=w203) -> ("Error Out"=w200:errorcluster, "Message"=w197:string)  [unwired: 2 in, 4 out]
          n44 = call <vilib>:"Clear Errors.vi"("error in (no error)"=w200, "specific error code to clear (0: all)"=1055) -> ("error out"=w202:errorcluster)  [unwired: 4 in, 1 out]
        }
        frame "jpeg", "jpg", "png", "tif", "tiff" {
          (unwired) T18 7 items=["Grayscale (U8)", "Grayscale (I16)", "Grayscale (SGL)", "Complex (CSG)", "RGB (U32)", "HSL (U32)", "RGB (U64)", "Grayscale (U16)"] ("Image Type")
          n45 = call "IMAQ GetFileInfo"("error in (no error)"=w214, "File Path"=w211) -> ("error out"=w212:errorcluster, "Image Type"=w213:T18)  [unwired: 3 in, 5 out]
          n46 = case shown="0, 1, 4, 7" w213 {
            tunnel: w212 -> [w217 w227 w246]
            tunnel: w211 -> [_ w225 w245]
            tunnel: [w216 w228 w244] -> w210
            tunnel: [w217 w226 w243] -> w209
            tunnel: w208 -> [w216 w219 _]
            frame 2, Default {
              # "not supported"
              n47 = One Button Dialog(message="Unsupported Image File Format!") -> ()  [unwired: 1 in, 1 out]
              n48 = call "Play Error Sound.vi"() -> ()  [unwired: 27 in, 1 out]
            }
            frame 0, 1, 4, 7 {
              # "U8 or U16: Mask Image or White Light Image"
              n49 = call "Three Buttons Dialog Window.vi"("Window Title"="Single Image Type Selection", "Button 2 Text"="White Light", "Button 1 Text (OK)"="Mask", "Message"="What type of image is this?") -> ("3-button Dialog Output"=w220:T19)  [unwired: 7 in]
              n50 = case shown="\"Button 2\"" w220 {
                tunnel: [w229 w238 w240] -> w228
                tunnel: w227 -> [_ w237 w242]
                tunnel: [w230 w236 w239] -> w226
                tunnel: w225 -> [_ w235 w241]
                tunnel: w219 -> [w229 _ _]
                frame "Window Close", Default {
                  n51 = xnode "Error Ring"() -> ("error out"=w230:errorcluster)
                }
                frame "Button 1" {
                  # "Mask"
                  n52 = call "AlliGator Script Open Mask Image.vi"("Error In"=w237, "Image Path"=w235) -> ("Error Out"=w236:errorcluster, "Action List out"=w238:T10[])  [unwired: 8 in]
                }
                frame "Button 2" {
                  # "White Light"
                  n53 = call "AlliGator Script Open White Light Image.vi"("Error In"=w242, "Image Path"=w241) -> ("Error Out"=w239:errorcluster, "Action List out"=w240:T10[])  [unwired: 8 in]
                }
              }
            }
            frame 16 {
              # "I16 or RGB: white light image"
              n54 = call "AlliGator Script Open White Light Image.vi"("Error In"=w246, "Image Path"=w245) -> ("Error Out"=w243:errorcluster, "Action List out"=w244:T10[])  [unwired: 8 in]
            }
          }
        }
        frame "phplot" {
          n55 = Build Array(w253) -> (w252:path[])
          n56 = Bundle By Name(cluster=T10 {"AlliGator Q Event"=enum."Phasor Graph:Load Phasor Plot(s)", "Data"=variant} ("Alligator Atomic Action"), "Data"=w252) -> (w250:T10)
          n57 = Build Array(w250) -> (w248:T10[])
        }
        frame "cal" {
          n58 = Bundle By Name(cluster=T13 {"Load/Save"=FALSE, "File Path"=path ""}, "File Path"=w259) -> (w260:T13)
          n59 = Bundle By Name(cluster=T10 {"AlliGator Q Event"=enum."Calibration:Load/Save Phasor Calibration", "Data"=variant} ("Alligator Atomic Action"), "Data"=w260) -> (w257:T10)
          n60 = Build Array(w257) -> (w256:T10[])
        }
        frame "caln" {
          n61 = Bundle By Name(cluster=T13 {"Load/Save"=FALSE, "File Path"=path ""}, "File Path"=w268) -> (w269:T13)
          n62 = Bundle By Name(cluster=T10 {"AlliGator Q Event"=enum."Calibration:Load/Save Phasor Calibration Series", "Data"=variant} ("Alligator Atomic Action"), "Data"=w269) -> (w267:T10)
          n63 = Build Array(w267) -> (w265:T10[])
        }
        frame "calm" {
          n64 = Bundle By Name(cluster=T13 {"Load/Save"=FALSE, "File Path"=path ""}, "File Path"=w277) -> (w278:T13)
          n65 = Bundle By Name(cluster=T10 {"AlliGator Q Event"=enum."Calibration:Load/Save Phasor Calibration Map", "Data"=variant} ("Alligator Atomic Action"), "Data"=w278) -> (w276:T10)
          n66 = Build Array(w276) -> (w274:T10[])
        }
        frame "ref" {
          n67 = Bundle By Name(cluster=T10 {"AlliGator Q Event"=enum."Phasor Ratio:Load References", "Data"=variant} ("Alligator Atomic Action"), "Data"=w282) -> (w286:T10)
          n68 = Build Array(w286) -> (w284:T10[])
        }
      }
      n69 = case shown="False" w46 {
        tunnel: w38 -> [_ w77]
        tunnel: w51 -> [w73 w76]
        tunnel: [w72 w76] -> w41
        tunnel: [w71 w77] -> w50
        tunnel: w48 -> [w70 _]
        tunnel: w47 -> [w69 _]
        tunnel: w32 -> [w68 _]
        tunnel: w31 -> [w67 _]
        tunnel: w33 -> [w66 _]
        frame False {
          # "Dataset"
          n70 = case shown="\"White Ligth Image\", \"Mask Image\"" w66 {
            selector: w66 -> [w74 _]
            tunnel: [w74 AlliGator_Displayed_Image."Sum of All Gates" ("Type of Displayed Image")] -> w65
            frame "Single Gate", Default {
            }
            frame "White Ligth Image", "Mask Image" {
            }
          }
          n71 = call "AlliGator Script_Open Single FLI Dataset.vi"("Type of Displayed Image"=w65, "FLI Dataset Type"=w69, "File Path"=w70, "Save Image with Overlay"=w68, "Error In"=w73, "Save Phasor Plot with Overlay"=w67) -> ("Action List out"=w71:T10[], "Error Out"=w72:errorcluster)  [unwired: 8 in]
        }
        frame True {
          # "not a dataset"
        }
      }
    }
    frame True {
      # "Folder: is it a Gate Folder or a Series?"
      n72 = call <userlib>:"List Directory__ogtk.vi"("error in (no error)"=w300, "directory path"=w301) -> ("error out"=w296:errorcluster, "directory names"=w294:string[], "file names"=w293:string[], "dup directory path"=w297:path)  [unwired: 2 in]
      n73 = Empty Array?(array=w293) -> (empty?=w298:bool)
      n74 = case shown="False" w298 {
        tunnel: w297 -> [w315 w414]
        tunnel: w296 -> [w314 w413]
        tunnel: [w311 w416] -> w299
        tunnel: [w310 w415] -> w295
        tunnel: w294 -> [w304 w418]
        tunnel: w293 -> [w307 _]
        tunnel: w292 -> [w306 w412]
        tunnel: w291 -> [w305 w411]
        tunnel: w289 -> [w302 _]
        frame False {
          # "files are present: are they gate images?"
          n75 = Empty Array?(array=w304) -> (empty?=w303:bool)
          n76 = call "Vision Toolkit Supported Files.vi"() -> ("Pattern String"=w316:string)  [unwired: 7 in, 1 out]
          n77 = call "Get Ordered List of Files.vi"("pattern"=w316, "Split string"="_Delay=", "Error In"=w314, "Folder Path"=w315) -> ("Error Out"=w312:errorcluster, "Folder Path dup"=w309:path, "Ordered File Paths"=w308:path[])  [unwired: 4 in, 1 out]
          n78 = Empty Array?(array=w308) -> (empty?=w313:bool)
          n79 = case shown="True" w313 {
            tunnel: w312 -> [w326 w335]
            tunnel: [w322 w336] -> w311
            tunnel: [w320 w334] -> w310
            tunnel: w309 -> [w321 w333]
            tunnel: w307 -> [_ w329]
            tunnel: w306 -> [w325 w332]
            tunnel: w305 -> [w324 w331]
            tunnel: w303 -> [_ w330]
            tunnel: w302 -> [w319 _]
            frame False {
              # "Images found: go for single gate image folder"
              n80 = case shown="\"White Ligth Image\", \"Mask Image\"" w319 {
                selector: w319 -> [w327 _]
                tunnel: [w327 AlliGator_Displayed_Image."Sum of All Gates" ("Type of Displayed Image")] -> w318
                frame "Single Gate", Default {
                }
                frame "White Ligth Image", "Mask Image" {
                }
              }
              n81 = call "AlliGator Script_Open Single FLI Dataset.vi"("Type of Displayed Image"=w318, "FLI Dataset Type"=AlliGator_FLI_Dataset_Type."Gate Image Folder", "File Path"=w321, "Save Image with Overlay"=w325, "Error In"=w326, "Save Phasor Plot with Overlay"=w324) -> ("Action List out"=w320:T10[], "Error Out"=w322:errorcluster)  [unwired: 8 in]
            }
            frame True {
              w338 = string[] ["hdf5", "sdt", "ptu", "bin", "dat"] ("pattern")
              (unwired) "*.hdf5;*.sdt;*.ptu;*.bin;;*.dat" ("pattern")
              # "not gate images: try valid datasets"
              n82 = for {
                tunnel: w329 -> [w410] mode=indexing
                tunnel: [w408] -> w341 mode=indexing
                n83 = String To Path(string=w410) -> (path=w409:path)
                n84 = call <vilib>:"Get File Extension.vi"("file"=w409) -> ("lowercase file extension"=w408:string)  [unwired: 6 in, 4 out]
              }
              n85 = for {
                shift-right: [w405] -> _
                shift-left: w341 -> [w407]
                tunnel: w338 -> [w406] mode=indexing
                tunnel: [w403] -> w340 mode=indexing
                n86 = call-poly <userlib>:"Filter 1D Array__ogtk.vi"("items to filter"=w406, "array"=w407) -> ("filtered item indices"=w404:i32[], "filtered array"=w405:string[])  [unwired: 4 in]
                n87 = Array Size(array=w404) -> (size(s)=w403:i32)
              }
              n88 = Array Max & Min(array=w340) -> (max value=w337:i32, max index (indices)=w339:i32)  [unwired: 2 out]
              n89 = case shown="0" w337 {
                tunnel: w339 -> [_ w384]
                tunnel: w338 -> [_ w383]
                tunnel: [w344 w369] -> w336
                tunnel: w335 -> [w347 w376]
                tunnel: [w348 w370] -> w334
                tunnel: w333 -> [w343 w368]
                tunnel: w332 -> [w346 w374]
                tunnel: w331 -> [w345 w373]
                tunnel: w330 -> [w342 _]
                tunnel: w329 -> [_ w367]
                frame 0 {
                  # "No valid file"
                  n90 = case shown="False" w342 {
                    tunnel: [w349 w362] -> w344
                    tunnel: [w350 _] -> w348
                    tunnel: w343 -> [w357 _]
                    tunnel: w347 -> [w355 _]
                    tunnel: w346 -> [w354 _]
                    tunnel: w345 -> [w353 _]
                    frame False {
                      # "subfolders are present: try folder of gate image folders"
                      n91 = Bundle(cluster=T16 {"Folder Selection Mode"=enum."Select Gate Folder", "Folder Path"=path ""} ("Folder Selection"), "Folder Selection Mode"=AlliGator_Select_Folder_Mode."Select Folder of Gate Folders", "Folder Path"=w357) -> (w359:T16)
                      n92 = Bundle By Name(cluster=T10 {"AlliGator Q Event"=enum."Files:Select Folder", "Data"=variant} ("Time-Gated Phasor Q Element"), "Data"=w359) -> (w356:T10)
                      n93 = call "AlliGator Post Loading Action List.vi"("Error In"=w355, "Save Phasor Plot with Overlay (F)"=w353, "Save Image with Overlay (F)"=w354, "Load Image only? (F)"=FALSE ("Load Image only?")) -> ("Error Out"=w349:errorcluster, "Action List"=w351:T10[])  [unwired: 6 in]
                      n94 = Build Array (concatenate)(w356, w351) -> (w350:T10[])
                    }
                    frame True {
                      # "No subfolders: invalid selection"
                      n95 = xnode "Error Ring"() -> ("error out"=w362:errorcluster)
                    }
                  }
                }
                frame 1, Default {
                  # "looks for the majority type"
                  n96 = Index Array(array=w383, index=w384) -> (element=w377:string)
                  n97 = case shown="\"bin\"" w377 {
                    tunnel: [_ AlliGator_Select_Folder_Mode."Select Folder of HDF5 FLI Datasets" AlliGator_Select_Folder_Mode."Select Folder of .sdt FLI Datasets (Becker & Hickl)" AlliGator_Select_Folder_Mode."Select Folder of .ptu FLI Datasets (PicoQuant)" w396] -> w381
                    tunnel: w376 -> [_ w390 w392 w394 w398]
                    tunnel: [w385 w390 w392 w394 w397] -> w375
                    tunnel: w368 -> [_ _ _ _ w401]
                    tunnel: w367 -> [_ _ _ _ w402]
                    frame "", Default {
                      n98 = xnode "Error Ring"() -> ("error out"=w385:errorcluster)
                    }
                    frame "hdf5" {
                    }
                    frame "sdt" {
                    }
                    frame "ptu" {
                    }
                    frame "bin" {
                      n99 = Index Array(array=w402) -> (element=w400:string)  [unwired: 1 in]
                      n100 = Build Path(base path=w401, name or relative path=w400) -> (appended path=w399:path)
                      n101 = call "AlliGator Check .bin File Type.vi"("error in (no error)"=w398, "File Path"=w399) -> ("error out"=w397:errorcluster, "Folder Selection Mode"=w396:T17)  [unwired: 6 in, 2 out]
                    }
                  }
                  n102 = Bundle(cluster=T16 {"Folder Selection Mode"=enum."Select Gate Folder", "Folder Path"=path ""} ("Folder Selection"), "Folder Selection Mode"=w381, "Folder Path"=w368) -> (w380:T16)
                  n103 = call "AlliGator Post Loading Action List.vi"("Error In"=w375, "Save Phasor Plot with Overlay (F)"=w373, "Save Image with Overlay (F)"=w374, "Load Image only? (F)"=FALSE ("Load Image only?")) -> ("Error Out"=w369:errorcluster, "Action List"=w372:T10[])  [unwired: 6 in]
                  n104 = Bundle By Name(cluster=T10 {"AlliGator Q Event"=enum."Files:Select Folder", "Data"=variant} ("Time-Gated Phasor Q Element"), "Data"=w380) -> (w378:T10)
                  n105 = Build Array (concatenate)(w378, w372) -> (w370:T10[])
                }
              }
            }
          }
        }
        frame True {
          # "No valid file: try folder of gate image folders"
          n106 = Empty Array?(array=w418) -> (empty?=w417:bool)
          n107 = case shown="False" w417 {
            tunnel: [w419 w432] -> w416
            tunnel: [w420 _] -> w415
            tunnel: w414 -> [w427 _]
            tunnel: w413 -> [w425 _]
            tunnel: w412 -> [w424 _]
            tunnel: w411 -> [w423 _]
            frame False {
              # "subfolders are present: try folder of gate image folders"
              n108 = Bundle(cluster=T16 {"Folder Selection Mode"=enum."Select Gate Folder", "Folder Path"=path ""} ("Folder Selection"), "Folder Selection Mode"=AlliGator_Select_Folder_Mode."Select Folder of Gate Folders", "Folder Path"=w427) -> (w429:T16)
              n109 = Bundle By Name(cluster=T10 {"AlliGator Q Event"=enum."Files:Select Folder", "Data"=variant} ("Time-Gated Phasor Q Element"), "Data"=w429) -> (w426:T10)
              n110 = call "AlliGator Post Loading Action List.vi"("Error In"=w425, "Save Phasor Plot with Overlay (F)"=w423, "Save Image with Overlay (F)"=w424, "Load Image only? (F)"=FALSE ("Load Image only?")) -> ("Error Out"=w419:errorcluster, "Action List"=w421:T10[])  [unwired: 6 in]
              n111 = Build Array (concatenate)(w426, w421) -> (w420:T10[])
            }
            frame True {
              # "No subfolders: invalid selection"
              n112 = xnode "Error Ring"() -> ("error out"=w432:errorcluster)
            }
          }
        }
      }
    }
  }
  "AlliGator Q Elements out" <- w19
  "error out" <- w20
  "Message" <- w5
  "Script out" <- w2
